vi "load_tdms.vi"(8 "error in (no error)":errorcluster, 11 "Path":path) -> (0 "error out":errorcluster, 3 "Data":dbl[](array[numeric]))   [LabVIEW 2024]
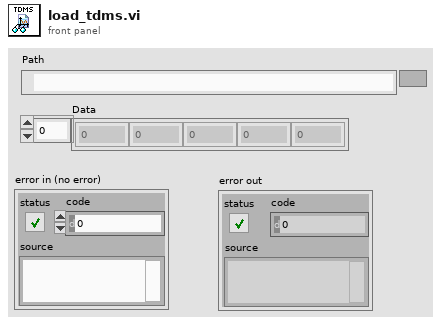
[diagram p1: front panel]
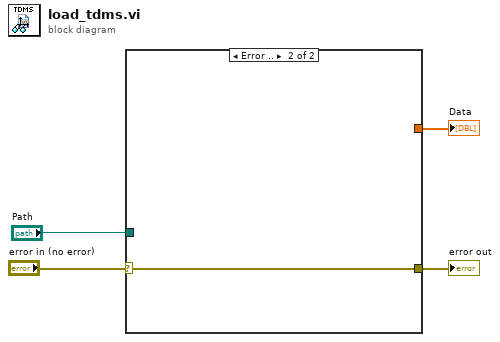
[diagram p0: block diagram]
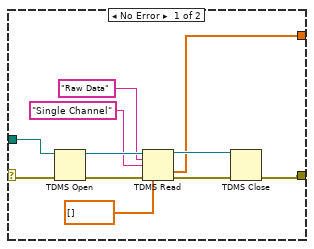
[diagram p2: hidden frame]
diagram:
  n1 = case shown="Error .." "error in (no error)" {
    selector: "error in (no error)" -> [w15 w16]
    tunnel: [w9 w16] -> w3
    tunnel: "Path" -> [w14 _]
    tunnel: [w6 _] -> w1
    frame No Error {
      n2 = TDMS Open(8:w15, 11:w14) -> (0:w12:errorcluster, 3:w13:refnum<k34>)  [unwired: 5 in]
      n3 = TDMS Read(0:w13, 5:"Raw Data" ("group name in"), 7:"Single Channel" ("group name in"), 11:w12, 12:dbl[] []) -> (4:w11:refnum<k34>, 10:w6:dbl[], 15:w10:errorcluster)  [unwired: 3 in, 3 out]
      n4 = TDMS Close(8:w10, 11:w11) -> (0:w9:errorcluster)  [unwired: 1 out]
    }
    frame Error {
    }
  }
  "error out" <- w3
  "Data" <- w1
